vi "Read Initial Data to String.vi"() -> (0 "Data":string)   [LabVIEW 2012]
doc: "The Basic Serial Read and Write example performs a Serial Port Read, a Serial Port Write, or a combination of these actions. The user selects the actions (read or write) on the front panel. If both are selected, the VI will write the data first, read data, and then close the VISA session that is opened to the port. This VI will wait until the specified number of bytes is received at the port or until a termination character is read.\n\nINSTRUCTIONS:\n1) Select the serial resource and configuration parameters (baud rate, data bits, parity, stop bits, flow control).\n2) Select the operations to be performed. \n3) Connect the serial port to your device. If no device is available, perform a loopback test by doing one of the following. Short pins 2 and 3 on a RS-232 cable or short pin 4 to pin 8 and pin 5 to pin 9 on a RS-485/422 cable. \n4) Run the VI to see the data read. (The \"read string\" will match the \"string to write\" if a loopback test was performed.)\n\nNote: The parameters set for the serial port must match the parameters of the connected instrument or device. In this example, the bytes to read parameter specifies the number of bytes that the serial port reads. If there were more bytes at the port than the number specified in bytes to read, those bytes would not be read. Also, if you specify to read more bytes than the number of bytes actually read, you might receive a timeout error message.\n\nOn the block diagram, the Configure Serial Port VI sets the configuration parameters. The front panel displays the controls used to configure the basic parameters, such as baud rate, data bits, and parity. Constants configure the other parameters the user probably does not need set. After the VISA Configure Serial Port VI opens the VISA session and configures the port, the VI passes the VISA resource name to other VIs that perform operations on that VISA resource. The VISA Write function sends a command to the serial device and the VISA Read function returns data based on the command. The VISA Close function then closes the reference to the serial device. It is important to close the reference; otherwise communication through with that port through protocols other than VISA might not be possible."
uses:
  Correlator port.vi
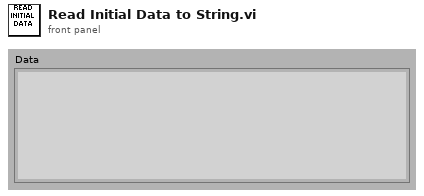
[diagram p1: front panel]
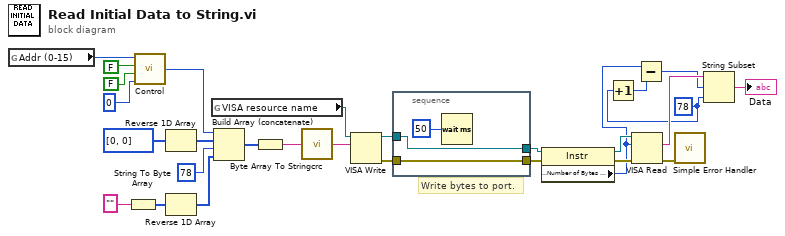
[diagram p0: block diagram]
diagram:
  w4 = 78 ("length (rest)")
  # "Write bytes to port."
  n1 = global read "Correlator port.vi" "Addr (0-15)"() -> (w8:i8)
  n2 = String To Byte Array(string="" ("Data")) -> (unsigned byte array=w14:u8[])
  n3 = call "Control.vi"("Page"=i8 0, "Error"=FALSE, "Write"=FALSE, "Addr"=w8) -> ("Control Byte"=w19:u32)
  n4 = Reverse 1D Array(array=i8[] [0, 0] ("Offset")) -> (reversed array=w17:i8[])
  n5 = Reverse 1D Array(array=w14) -> (reversed array=w13:u8[])
  n6 = global read "Correlator port.vi" "VISA resource name"() -> (w9:refnum<visa-resource-name>)
  n7 = Build Array (concatenate)(w19, w17, u8 78 ("Length"), w13) -> (w12:u32[])
  n8 = Byte Array To String(unsigned byte array=w12) -> (string=w11:string)
  n9 = call "crc.vi"("Input string"=w11) -> ("Output (with crc)"=w10:string)
  n10 = VISA Write(VISA resource name=w9, write buffer=w10) -> (VISA resource name out=w26:refnum<visa-resource-name>, error out=w28:errorcluster)  [unwired: 1 in, 1 out]
  n11 = stacked-sequence {
    tunnel: w28 -> [w31]
    tunnel: [w31] -> w27
    tunnel: w26 -> [w30]
    tunnel: [w30] -> w25
    frame #0 {
      n12 = Wait (ms)(milliseconds to wait=u32 50 ("delay before read (ms)")) -> ()  [unwired: 1 out]
    }
  }
  n13 = property class="Instr"(reference=w25, error in=w27) -> (reference out=w7:refnum<visa-resource-name>, error out=w6:errorcluster, "Serial Settings:Number of Bytes at Serial Port"=w2:u32)
  n14 = Increment(x=w4) -> (x+1=w3:i32)
  n15 = VISA Read(VISA resource name=w7, byte count=w2, error in (no error)=w6) -> (read buffer=w24:string, error out=w5:errorcluster)  [unwired: 2 out]
  n16 = Subtract(x=w2, y=w3) -> (x-y=w1:u32)
  n17 = call <vilib>:"Simple Error Handler.vi"("error in (no error)"=w5) -> ()  [unwired: 1 in, 8 out]
  n18 = String Subset(string=w24, offset (0)=w1, length (rest)=w4) -> (substring=→"Data":string)
